vi "sv_Check Data Valid [Weighting].vi"(6 "reset (in)":bool, 8 "error in (no error)":errorcluster, 9 "weighting":T1 items=["Linear", "A-weighting", "B-weighting", "C-weighting", "ITU-R 468-4", "Dolby", "CCITT", "C-message", "Wb", "Wc", "Wd", "We", "Wf", "Wh", "Wj", "Wk", "Wm", "AES17 20 kHz lowpass", "AES17 40 kHz lowpass", "AES17 20 kHz highpass", "AES17 40 kHz highpass"], 11 "signal in [X]":waveform(dbl)={"t0"=timestamp(0 s since 1904-01-01), "dt"=1.953125e-05, "Y"=[]}) -> (0 "error out":errorcluster, 1 "weighting":T1 items=["Linear", "A-weighting", "B-weighting", "C-weighting", "ITU-R 468-4", "Dolby", "CCITT", "C-message", "Wb", "Wc", "Wd", "We", "Wf", "Wh", "Wj", "Wk", "Wm", "AES17 20 kHz lowpass", "AES17 40 kHz lowpass", "AES17 20 kHz highpass", "AES17 40 kHz highpass"], 3 "signal out [X]":waveform(dbl)={"t0"=timestamp(0 s since 1904-01-01), "dt"=1.953125e-05, "Y"=[]}, 4 "reset (out)":bool)   [LabVIEW 2017]
uses:
  <vilib>/addons/_NISVFA/_Shared subVIs/Controls/svc_Weighting Filter Text Ring.ctl
  <vilib>/addons/_NISVFA/_Shared subVIs/Common/svc_Check for Waveform Parameter Continuity (no state).vi
  <vilib>/addons/_NISVFA/_Shared subVIs/Common/svc_Get SV Channel Info.vi
  <vilib>/addons/_NISVFA/_Shared subVIs/Common/svc_Engineering Units to Unit Label.vi
  <vilib>/addons/_NISVFA/_Shared subVIs/Common/svc_Unit Label to Engineering Units.vi
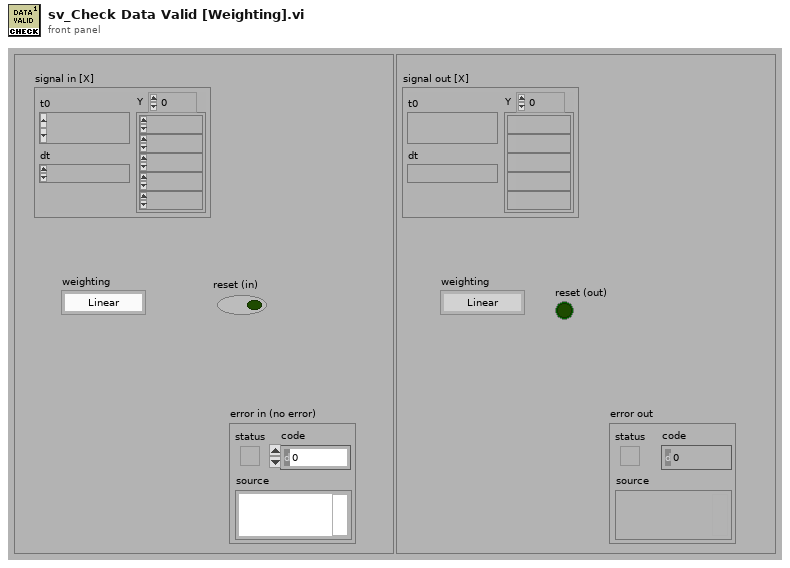
[diagram p1: front panel]
types:
  T1 = typedef "svc_Weighting Filter Text Ring.ctl" = u16
  T2 = cluster{"dt":bool, "t0 continuity":bool, "array length":bool, "channel info":bool, "name":bool}
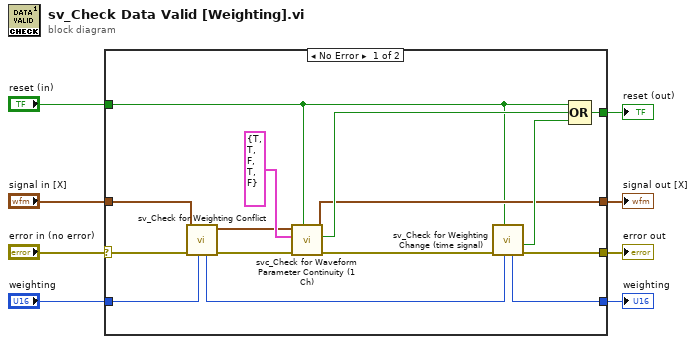
[diagram p0: block diagram]
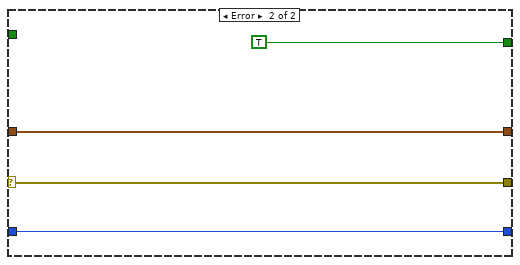
[diagram p2: hidden frame]
diagram:
  n1 = case shown="No Error" "error in (no error)" {
    selector: "error in (no error)" -> [w21 w27]
    tunnel: "weighting" -> [w23 w24]
    tunnel: "signal in [X]" -> [w11 w26]
    tunnel: [w22 TRUE ("t0 changed")] -> w5
    tunnel: [w19 w27] -> w4
    tunnel: [w13 w26] -> w3
    tunnel: "reset (in)" -> [w9 _]
    tunnel: [w20 w24] -> w1
    frame No Error {
      n2 = call <vilib>:"sv_Check for Weighting Conflict.vi"("weighting"=w23, "error in (no error)"=w21, "scaled signal [EU]"=w11) -> ("error out"=w15:errorcluster, "scaled signal [EU]"=w12:waveform(dbl), "dup weighting"=w10:T1)  [unwired: 6 in]
      n3 = call <vilib>:"svc_Check for Waveform Parameter Continuity (1 Ch).vi"("restart averaging (F)"=w9, "error in (no error)"=w15, "checks for channel parameter change"=T2 {"dt"=TRUE, "t0 continuity"=TRUE, "array length"=FALSE, "channel info"=TRUE, "name"=FALSE}, "scaled signal [EU]"=w12) -> ("error out"=w14:errorcluster, "waveform parameter changed"=w16:bool, "dup scaled signal [EU]"=w13:waveform(dbl))  [unwired: 2 in, 3 out]
      n4 = call <vilib>:"sv_Check for Weighting Change (time signal).vi"("weighting"=w10, "reset (in)"=w9, "error in (no error)"=w14) -> ("error out"=w19:errorcluster, "weighting has changed"=w18:bool, "dup weighting"=w20:T1)  [unwired: 6 in]
      n5 = Compound Arithmetic op=OR(w9, w16, w18) -> (w22:bool)
    }
    frame Error {
    }
  }
  "error out" <- w4
  "signal out [X]" <- w3
  "reset (out)" <- w5
  "weighting" <- w1
